vi "Data Processing Loop.vi"(8 "Error In":errorcluster, 11 "TopLevel":T1) -> (0 "Error Out":errorcluster)   [LabVIEW 2011]
uses:
  Controls/Top Level Control.ctl
  <vilib>/NI/AMC/Message Queue.ctl
  <vilib>/NI/AMC/Message.ctl
  <vilib>/NI/Tools/Keyed Array/KeyedArray.ctl
  Controls/ListBox Test Record.ctl
  Controls/DVR of CSV Tests Data.ctl
  Controls/CSVs Tests Data.ctl
  Controls/Test Column Data.ctl
  Controls/Options DVR.ctl
  Controls/Options.ctl
  Controls/DPL Request.ctl
  <vilib>/NI/AMC/Read Termination Message.vi
  <vilib>/NI/AMC/Create Single Message.vi
  <vilib>/NI/AMC/Update Message Routing Info.vi
  Create Graph Data.vi
  Create Failure Data.vi
  Create Log Data.vi
  <vilib>/NI/AMC/Globals.vi
  Analysis/Read Actual Values From Log File.vi
  <vilib>/NI/AMC/Send Message.vi
  Analysis/Read All Actual Values From Log File.vi
  <vilib>/Utility/libraryn.llb/Get File Extension.vi
  <vilib>/NI/AMC/AMC.lvlib
  <vilib>/NI/Tools/Keyed Array/Tools_KeyedArray.lvlib
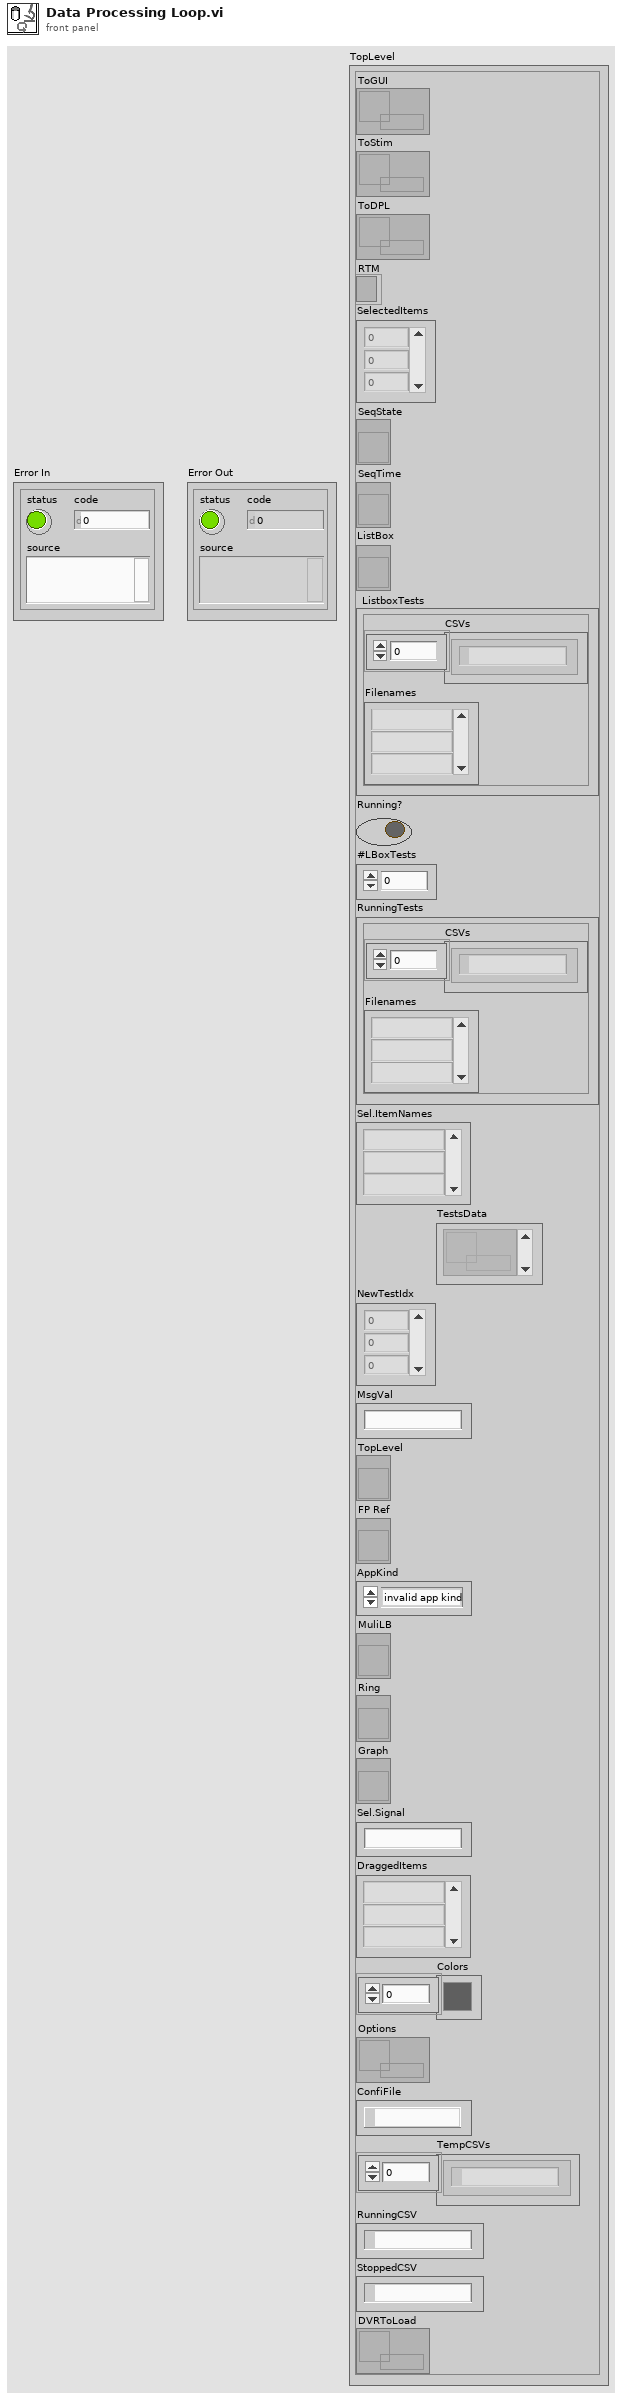
[diagram p1: front panel]
types:
  T1 = typedef "Top Level Control.ctl" = cluster{"ToGUI":T2, "ToStim":T2, "ToDPL":T2, "RTM":refnum<k9>, "SelectedItems":i32[], "SeqState":refnum<vi>, "SeqTime":refnum<vi>, "ListBox":refnum<vi>, "ListboxTests":T3, "Running?":bool, "#LBoxTests":i32, "RunningTests":T3, "Sel.ItemNames":string[], "TestsData":T4[], "NewTestIdx":i32[], "MsgVal":string, "TopLevel":refnum<vi>, "FP Ref":refnum<vi>, "AppKind":enum32{"invalid app kind", "Development System", "Run Time System", "Student Edition", "Embedded LabVIEW", "Evaluation", "Custom"}, "MuliLB":refnum<vi>, "Ring":refnum<vi>, "Graph":refnum<vi>, "Sel.Signal":string, "DraggedItems":string[], "Colors":u32[], "Options":T5, "ConfiFile":path, "TempCSVs":path[], "RunningCSV":path, "StoppedCSV":path, "DVRToLoad":T4}
  T2 = typedef "AMC.lvlib/Message Queue.ctl" = refnum<queue>
  T3 = typedef "ListBox Test Record.ctl" = cluster{"CSVs":path[], "Filenames":string[]}
  T4 = typedef "DVR of CSV Tests Data.ctl" = refnum<data-value>
  T5 = typedef "Options DVR.ctl" = refnum<data-value>
  T6 = typedef "DPL Request.ctl" = cluster{"TestRec":T4, "Signal":string}
  T7 = typedef "Test Data Record.ctl" = cluster{"Graph Data":dbl[][], "MuliLB Data":string[][]}
  T8 = typedef "Options.ctl" = cluster{"Logging?":bool, "TimeStamp?":bool, "LogInCSVDir?":bool, "LogDir":path}
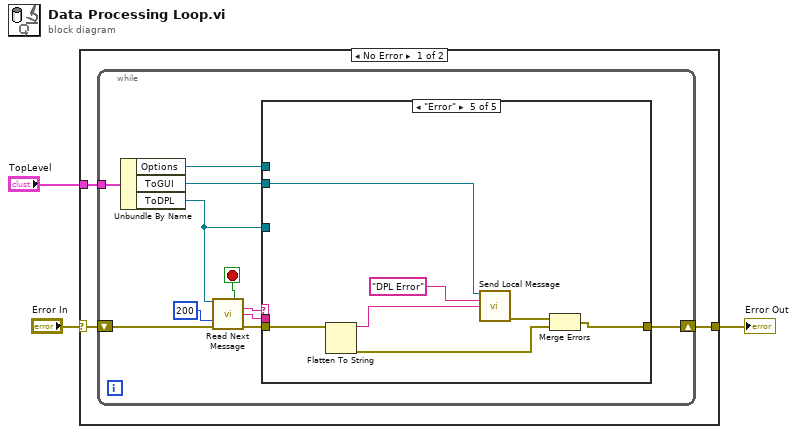
[diagram p0: block diagram]
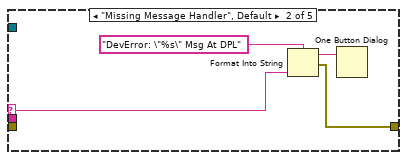
[diagram p3: hidden frame]
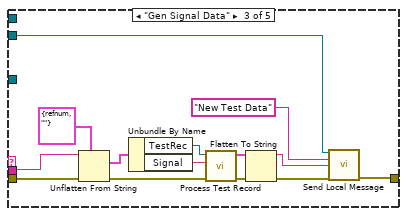
[diagram p4: hidden frame]
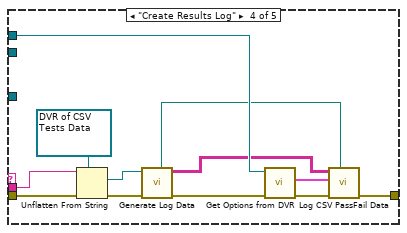
[diagram p5: hidden frame]
diagram:
  n1 = case shown="No Error" "Error In" {
    selector: "Error In" -> [w5 w56]
    tunnel: [w4 w56] -> w1
    tunnel: "TopLevel" -> [w6 _]
    frame No Error {
      n2 = while {
        tunnel: w6 -> [w17]
        shift-right: [w8] -> w4
        shift-left: w5 -> [w16]
        stop <- w14 stop-if-true
        n3 = Unbundle By Name(w17) -> ("Options"=w7:T5, "ToGUI"=w9:T2, "ToDPL"=w10:T2)
        n4 = call <vilib>:"Read Next Message.vi"("message queue in"=w10, "timeout (1 ms)"=200 ("timeout (1ms)"), "error in"=w16) -> ("exit process?"=w14:bool, "message name"=w13:string, "message value"=w11:string, "error out"=w12:errorcluster)  [unwired: 5 in, 4 out]
        n5 = case shown="\"Error\"" w13 {
          selector: w13 -> [_ w19 _ _ _]
          tunnel: w12 -> [w18 _ w36 w48 w53]
          tunnel: w11 -> [_ _ w34 w47 _]
          tunnel: w10 -> [_ _ _ _ _]
          tunnel: w9 -> [_ _ w32 _ w49]
          tunnel: [w18 w20 w28 w40 w50] -> w8
          tunnel: w7 -> [_ _ _ w46 _]
          frame "", "Exit" {
          }
          frame "Missing Message Handler", Default {
            n6 = Format Into String(format string="DevError: \"%s\" Msg At DPL" ("message"), w19) -> (resulting string=w22:string, error out=w20:errorcluster)  [unwired: 2 in]
            n7 = One Button Dialog(message=w22) -> ()  [unwired: 2 out]
          }
          frame "Gen Signal Data" {
            n8 = Unflatten From String(type=T6 {"TestRec"=refnum, "Signal"=""} ("DPL Request"), binary string=w34, error in (no error)=w36) -> (value=w25:T6, error out=w33:errorcluster)  [unwired: 2 in, 1 out]
            n9 = Unbundle By Name(w25) -> ("TestRec"=w23:T4, "Signal"=w24:string)
            n10 = call "Process Test Record.vi"("error in (no error)"=w33, "Signal"=w24, "TestRec"=w23) -> ("error out"=w31:errorcluster, "Data Record"=w30:T7)  [unwired: 7 in]
            n11 = Flatten To String(anything=w30, error in (no error)=w31) -> (data string=w26:string, error out=w29:errorcluster)  [unwired: 2 in, 1 out]
            n12 = call <vilib>:"Send Local Message.vi"("message queue in"=w32, "message name"="New Test Data" ("Message Name"), "message value"=w26, "error in"=w29) -> ("error out"=w28:errorcluster)  [unwired: 9 in, 2 out]
          }
          frame "Create Results Log" {
            n13 = Unflatten From String(type=T4 refnum ("TestRec"), binary string=w47, error in (no error)=w48) -> (value=w43:T4, error out=w44:errorcluster)  [unwired: 2 in, 1 out]
            n14 = call "Generate Log Data.vi"("error in (no error)"=w44, "TestRec"=w43) -> ("error out"=w42:errorcluster, "Log Data"=w38:string[][], "CsvPath"=w39:path)  [unwired: 7 in]
            n15 = call "Get Options from DVR.vi"("Error In"=w42, "Options DVR"=w46) -> ("Error Out"=w41:errorcluster, "Options"=w37:T8)  [unwired: 7 in, 1 out]
            n16 = call "Log CSV PassFail Data.vi"("Source CSV Path"=w39, "Error In"=w41, "Options"=w37, "Log Data"=w38) -> ("Error Out"=w40:errorcluster)  [unwired: 7 in]
          }
          frame "Error" {
            n17 = Flatten To String(anything=w53) -> (data string=w55:string, error out=w51:errorcluster)  [unwired: 3 in, 1 out]
            n18 = call <vilib>:"Send Local Message.vi"("message queue in"=w49, "message name"="DPL Error" ("Message Name"), "message value"=w55) -> ("error out"=w52:errorcluster)  [unwired: 10 in, 2 out]
            n19 = Merge Errors(w52, w51) -> (w50:errorcluster)
          }
        }
      }
    }
    frame Error {
    }
  }
  "Error Out" <- w1
